vi "Check Keys.vi"(7 "Time":timestamp, 11 "Sorted Data in":T1) -> (1 "codelapse":bool, 3 "Sorted Data Out":T1)   [LabVIEW 2013]
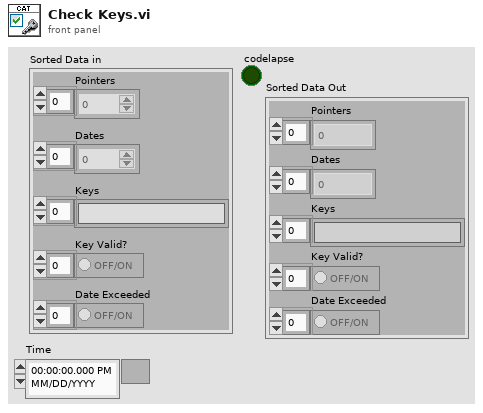
[diagram p1: front panel]
types:
  T1 = cluster{"Pointers":i32[], "Dates":dbl[], "Keys":string[], "Key Valid?":bool[], "Date Exceeded":bool[]}
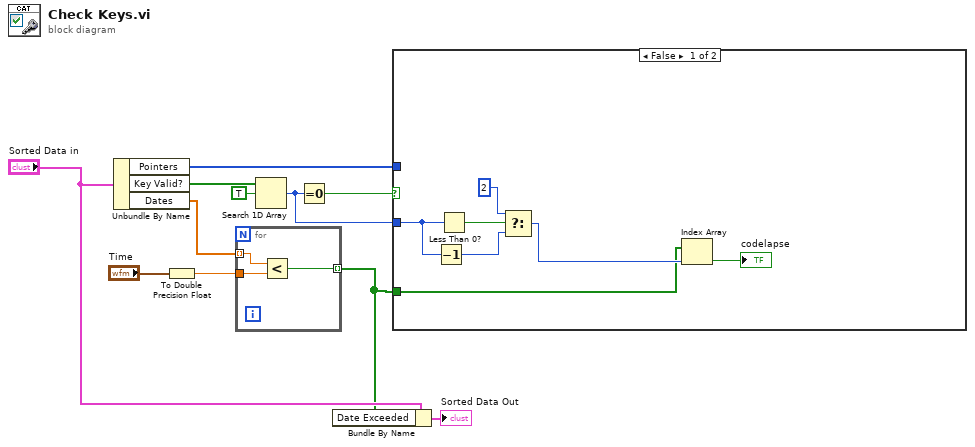
[diagram p0: block diagram]
diagram:
  n1 = Unbundle By Name("Sorted Data in") -> ("Pointers"=w3:i32[], "Key Valid?"=w8:bool[], "Dates"=w5:dbl[])
  n2 = To Double Precision Float(number="Time") -> (double precision float=w4:dbl)
  n3 = for {
    tunnel: w5 -> [w14] mode=indexing
    tunnel: w4 -> [w13]
    tunnel: [w12] -> w1 mode=indexing
    n4 = Less?(x=w14, y=w13) -> (x < y?=w12:bool)
  }
  n5 = Search 1D Array(1D array=w8, element=TRUE) -> (index of element=w2:i32)  [unwired: 1 in]
  n6 = Equal To 0?(x=w2) -> (x = 0?=w6:bool)
  n7 = Bundle By Name(cluster="Sorted Data in", "Date Exceeded"=w1) -> (→"Sorted Data Out":T1)
  n8 = case shown="False" w6 {
    tunnel: w3 -> [_ _]
    tunnel: w2 -> [w19 _]
    tunnel: w1 -> [w16 _]
    frame False {
      n9 = Decrement(x=w19) -> (x-1=w18:i32)
      n10 = Less Than 0?(x=w19) -> (x < 0?=w21:bool)
      n11 = Select(t=2, s=w21, f=w18) -> (s? t:f=w17:i32)
      n12 = Index Array(array=w16, index=w17) -> (element=→"codelapse":bool)
    }
    frame True {
    }
  }
